vi "Compute LO1 Frequencies with Formula.vi"(8 "error in (no error)":errorcluster, 9 "Spacing":dbl=500000000.0 format="%#_6p", 10 "Stop Frequency":dbl=6000000000.0 format="%#_6p", 11 "Start Frequency":dbl=4000000000.0 format="%#_6p") -> (0 "error out":errorcluster, 1 "Number of Records":i32, 2 "LO1 Frequencies":dbl[](array[numeric]) format="%#_6p", 3 "Carrier Frequencies":dbl[](array[numeric]) format="%#_6p")   [LabVIEW 2017]
uses:
  <vilib>/Analysis/1siggen.llb/Ramp Pattern by Delta.vi
  <vilib>/Analysis/NI_AALBase.lvlib
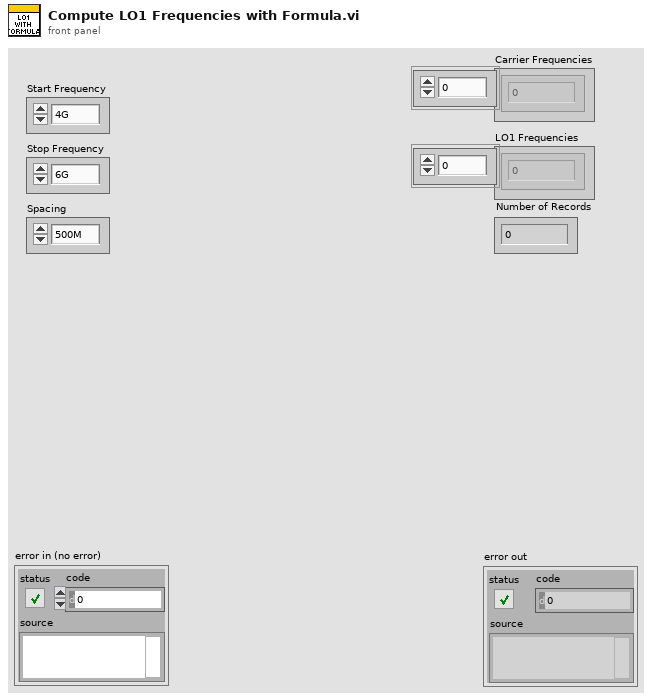
[diagram p1: front panel]
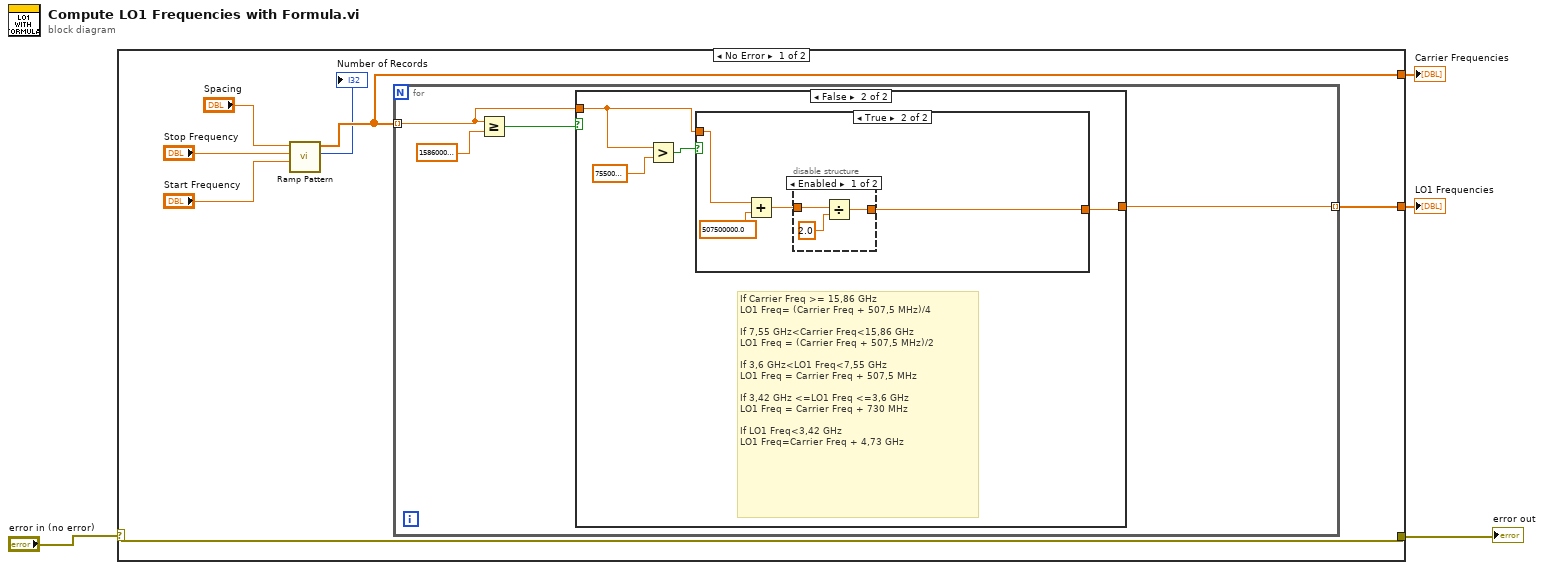
[diagram p0: block diagram]
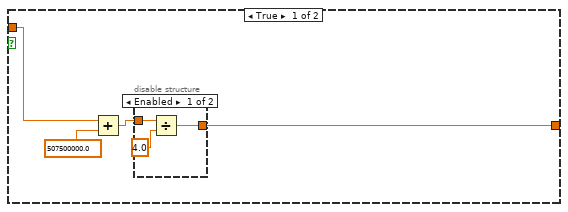
[diagram p2: hidden frame]
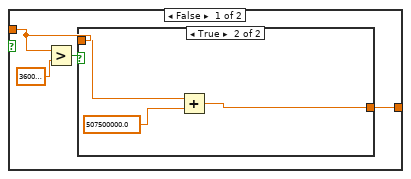
[diagram p4: hidden frame]
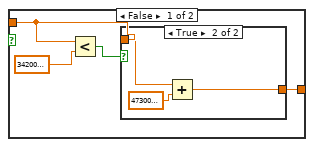
[diagram p5: hidden frame]
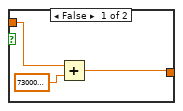
[diagram p6: hidden frame]
diagram:
  n1 = case shown="No Error" "error in (no error)" {
    selector: "error in (no error)" -> [w10 w53]
    tunnel: [w10 w53] -> w3
    tunnel: [w11 _] -> w2
    tunnel: [w6 _] -> w1
    frame No Error {
      n2 = call-poly <vilib>:"Ramp Pattern.vi"("start"="Start Frequency", "end"="Stop Frequency", "delta"="Spacing") -> ("samples"=→"Number of Records":i32, "Ramp Pattern"=w6:dbl[])  [unwired: 6 in, 1 out]
      n3 = for {
        tunnel: [w14] -> w11 mode=indexing
        tunnel: w6 -> [w13] mode=indexing
        n4 = Greater Or Equal?(x=w13, y=15860000000.0) -> (x >= y?=w12:bool)
        n5 = case shown="False" w12 {
          tunnel: [w17 w26] -> w14
          tunnel: w13 -> [w16 w25]
          frame True {
            n6 = Add(x=w16, y=507500000.0) -> (x+y=w18:dbl)
            n7 = disable-structure shown="Enabled" {
              disable-tunnel: w18 -> [w22 w23]
              disable-tunnel: [w20 w23] -> w17
              frame Enabled {
                n8 = Divide(x=w22, y=4.0) -> (x/y=w20:dbl)
              }
              frame Disabled {
              }
            }
          }
          frame False {
            # "If Carrier Freq >= 15,86 GHz\nLO1 Freq= (Carrier Freq + 507,5 MHz)/4\n\nIf 7,55 GHz<Carrier Freq<15,86 GHz\nLO1 Freq = (Carrier Freq + 507,5 MHz)/2\n\nIf 3,6 GHz<LO1 Freq<7,55 GHz\nLO1 Freq = Carrier Freq + 507,5 MHz\n\nIf 3,42 GHz <=LO1 Freq <=3,6 GHz \nLO1 Freq = Carrier Freq + 730 MHz\n\nIf LO1 Freq<3,42 GHz\nLO1 Freq=Carrier Freq + 4,73 GHz"
            n9 = Greater?(x=w25, y=7550000000.0) -> (0:w24:bool)
            n10 = case shown="True" w24 {
              tunnel: [w30 w46] -> w26
              tunnel: w25 -> [w29 w45]
              frame False {
                n11 = Greater?(x=w29, y=3600000000.0) -> (0:w28:bool)
                n12 = case shown="True" w28 {
                  tunnel: [w33 w43] -> w30
                  tunnel: w29 -> [w34 w42]
                  frame False {
                    n13 = Less?(x=w34, y=3420000000.0) -> (x < y?=w32:bool)
                    n14 = case shown="True" w32 {
                      tunnel: w34 -> [w36 w39]
                      tunnel: [w37 w40] -> w33
                      frame False {
                        n15 = Add(x=w36, y=730000000.0) -> (x+y=w37:dbl)
                      }
                      frame True {
                        n16 = Add(x=w39, y=4730000000.0) -> (x+y=w40:dbl)
                      }
                    }
                  }
                  frame True {
                    n17 = Add(x=w42, y=507500000.0) -> (x+y=w43:dbl)
                  }
                }
              }
              frame True {
                n18 = Add(x=w45, y=507500000.0) -> (x+y=w47:dbl)
                n19 = disable-structure shown="Enabled" {
                  disable-tunnel: w47 -> [w51 w52]
                  disable-tunnel: [w49 w52] -> w46
                  frame Enabled {
                    n20 = Divide(x=w51, y=2.0) -> (x/y=w49:dbl)
                  }
                  frame Disabled {
                  }
                }
              }
            }
          }
        }
      }
    }
    frame Error {
    }
  }
  "error out" <- w3
  "LO1 Frequencies" <- w2
  "Carrier Frequencies" <- w1
